vi "Enum.vi"(8 "error in":errorcluster, 11 "Enum":enum16{"A", "B", "C"}(ring)) -> (0 "error out":errorcluster, 3 "String":string)   [LabVIEW 2024]
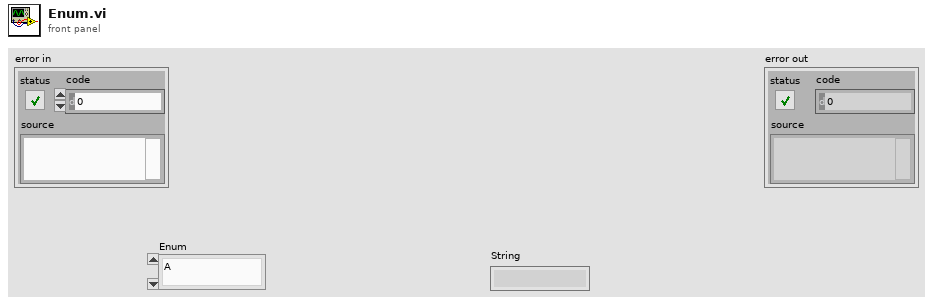
[diagram p1: front panel]
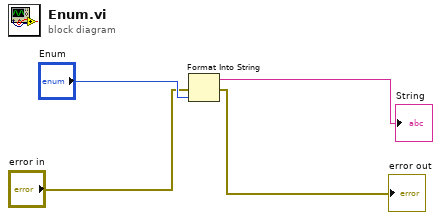
[diagram p0: block diagram]
diagram:
  n1 = Format Into String(error in="error in", "Enum") -> (resulting string=→"String":string, error out=→"error out":errorcluster)  [unwired: 2 in]
